vi "Global 1.vi"() -> ()   [LabVIEW 2013]
panel:
  out "Throttle Consistent":bool
  out "Throttles Connected":bool
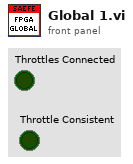
[diagram p1: front panel]
diagram:
